vi "RGBtoComplementar.vi"(1 "RGB":dbl[](array[numeric])) -> (0 "Complementar":u32(colorbox))   [LabVIEW 2013]
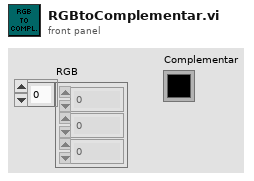
[diagram p1: front panel]
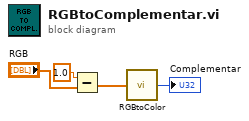
[diagram p0: block diagram]
diagram:
  n1 = Subtract(x=1.0, y="RGB") -> (x-y=w2:dbl[])
  n2 = call "RGBtoColor.vi"("RGB"=w2) -> ("Color"=→"Complementar":u32)
